vi "Example Two Stages.vi"() -> ()   [LabVIEW 2019]
uses:
  Class/Controller/Controller.lvclass
  <vilib>/Platform/TimedLoop/XDataNode/timing_clust.ctl
  <vilib>/Platform/TimedLoop/XDataNode/nitl_modes.ctl
  <vilib>/Platform/TimedLoop/XDataNode/wakeup.ctl
  <vilib>/platform/TimedLoop/XDataNode/XDataNode.xnode
  <vilib>/Platform/TimedLoop/XDataNode/XDNodeRunTimeDep.lvlib
panel:
  in  "Tab Control 2":enum32{"Motion", "Settings"}(tab)
  in  "Zero Output 2":bool
  in  "Go to Home 2":bool
  in  "Scan Right 2":bool
  in  "Scan Left 2":bool
  in  "Continue 2":bool
  in  "Stop 2":bool
  in  "Make Step Right 2":bool
  in  "Step Size \n[selected units] 2":dbl=1.0 format="%#.2f"
  in  "Make Step Left 2":bool
  in  "Desired Speed \n[1µm/s or 0,01deg /s] 2":dbl=10000.0 format="%#.2f"
  in  "Desired Position \n[selected units] 2":dbl format="%#.2f"
  in  "Find Index 2":bool
  in  "Reset 2":bool
  out "Desired Position\n[selected units] 2":dbl
  out "Encoder position \n[selected units] 2":dbl
  out "Waveform Chart 2":dbl(graph)=-0.078
  out "Status Info 2":T1
  out "StatusBits 2":T2
  out "Desired Position\n[selected units]":dbl
  out "Encoder position \n[selected units]":dbl
  in  "Tab Control":enum32{"Motion", "Settings"}(tab)
  in  "Zero Output":bool
  in  "Go to Home":bool
  in  "Scan Right":bool
  in  "Scan Left":bool
  in  "Continue":bool
  in  "Stop":bool
  in  "Make Step Right":bool
  in  "Step Size \n[selected units]":dbl=1.0 format="%#.2f"
  in  "Make Step Left":bool
  in  "Desired Speed \n[1µm/s or 0,01deg /s]":dbl=10000.0 format="%#.2f"
  in  "Desired Position \n[selected units]":dbl format="%#.2f"
  in  "Find Index":bool
  in  "Reset":bool
  out "error out":errorcluster
  in  "Working Units 2":string(combo)="1000000"
  in  "Working Units":string(combo)="1000000"
  out "StatusBits":T2
  out "Status Info":T1
  in  "Axis Resolution 2":string(combo)="312,5"
  in  "Axis Letter 2":string="Y"
  in  "Axis Resolution":string(combo)="312,5"
  in  "Axis Letter":string="X"
  in  "Baudrate":dbl=9600.0
  in  "COM Port":refnum<visa-resource-name>
  in  "Controller.lvclass":refnum<class "Controller.lvclass">
  out "Waveform Chart":dbl(graph)=-0.078
  in  "STOP PROGRAM":bool
  # "Visualization"
  # "Extra information"
  # "READ ME FIRST"
  # "Configuration"
  # "Stage 1"
  # "Driver 1"
  # "Stage 1"
  # "How to run:"
  # "BEFORE RUNNING:"
  # "1, Select COM Port"
  # "2. Select baudrate"
  # "3. For each axis:"
  # "3.1 Specify correct axis name (1 letter)"
  # "3.2 Specify correct resolution"
  # "4. Run VI"
  # "WHEN RUNNING, YOU HAVE TO FIRST PUSH \"FIND INDEX\" FOR EACH STAGE.\nThe stages will start moving and find its position. After that you can control the stages"
  # "Stage 2"
  # "NOTES: Do this only the first time"
  # "1. Replace the settings_default.txt file with\nthe file we provided on a USB stick."
  # "2.    Make sure there are no comments in the\nsettings_default.txt file. ONLY lines like: \"X:DPOS=100\" so NO \"%\" in front or at the end of the line."
  # "Position Information"
  # "STOP BUTTON"
  # "3.  In your settings_default.txt file:\nEvery line that contains SSPD or MSPD: multiply that value with:\n - 1000 for a lineair stage \n - 100 for a rotating stage"
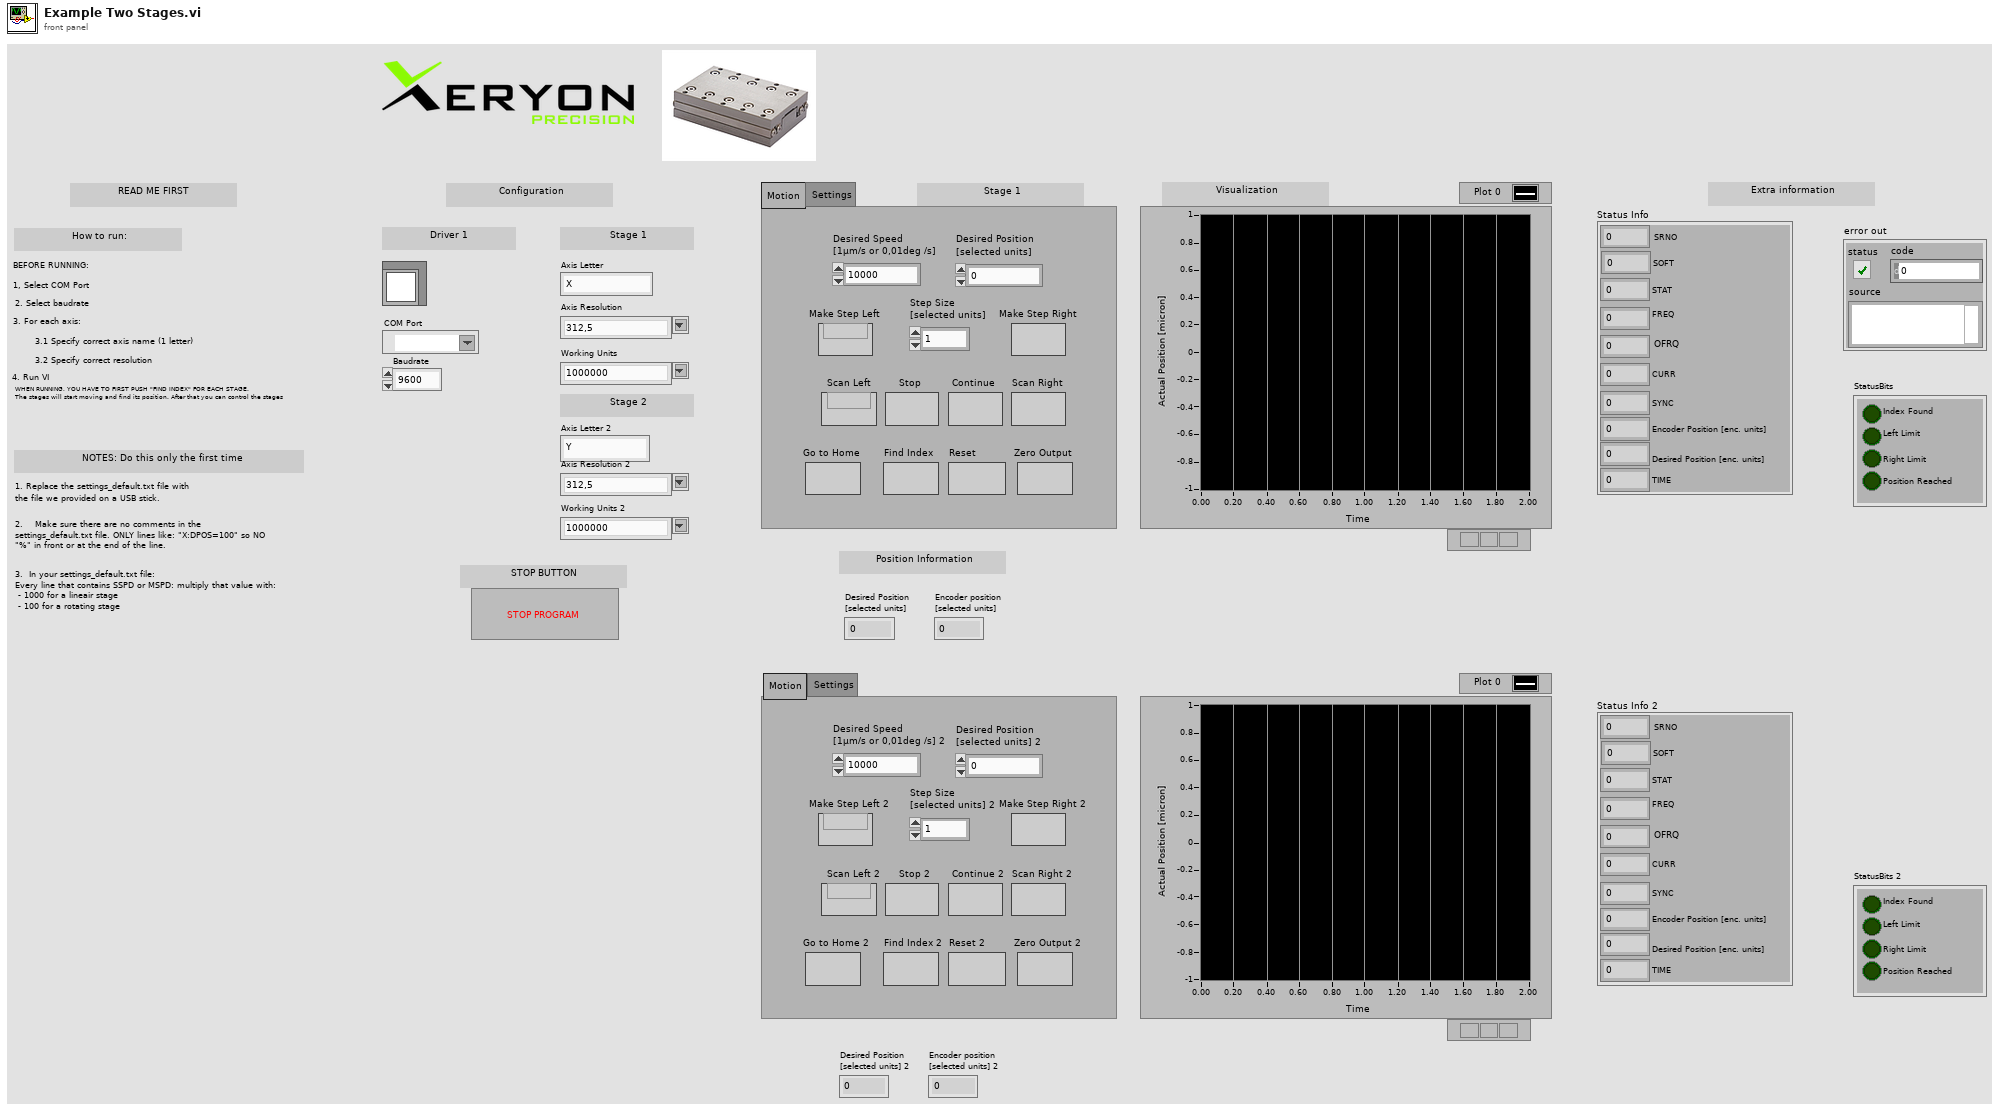
[diagram p1: front panel]
types:
  T1 = cluster{"SRNO":dbl, "SOFT":dbl, "STAT":dbl, "FREQ":dbl, "OFRQ":dbl, "CURR":dbl, "SYNC":dbl, "Encoder Position [enc. units]":dbl, "Desired Position [enc. units]":dbl, "TIME":dbl}
  T2 = cluster{"Index Found":bool, "Left Limit":bool, "Right Limit":bool, "Position Reached":bool}
  T3 = typedef "XDNodeRunTimeDep.lvlib/timing_clust.ctl" = cluster{"Expected End [f-1]":u64, "Actual End [f-1]":u64, "Finished Late? [f-1]":bool, "Expected End [i-1]":u64, "Actual End [i-1]":u64, "Finished Late? [i-1]":bool, "Expected Start [i]":u64, "Actual Start [i]":u64, "Expected Start [f]":u64, "Actual Start [f]":u64, "Source Name":string, "Structure Name":string, "Period":i64, "Deadline":i64, "Offset":i64, "Start":i64, "Priority":i32, "Timeout":i32, "Mode":T4, "Wakeup Reason":T5, "Error":errorcluster, "Source Type":string, "Secondary Source Type":string, "Global End Time":u64, "Global Start Time":u64, "Frame Duration":u64, "Iteration Duration":u64, "Assigned CPU":i32, "I/O Scan Engine Mode":u32}
  T4 = typedef "XDNodeRunTimeDep.lvlib/nitl_modes.ctl" = enum32{"No Change", "Process missed periods, maintain original phase", "Discard missed periods, maintain original phase", "Process missed periods, ignore original phase", "Discard missed periods, ignore original phase"}
  T5 = typedef "XDNodeRunTimeDep.lvlib/wakeup.ctl" = enum32{"Normal", "Aborted", "Asynchronous wakeup", "Timing source error", "Timed loop error", "Timeout"}
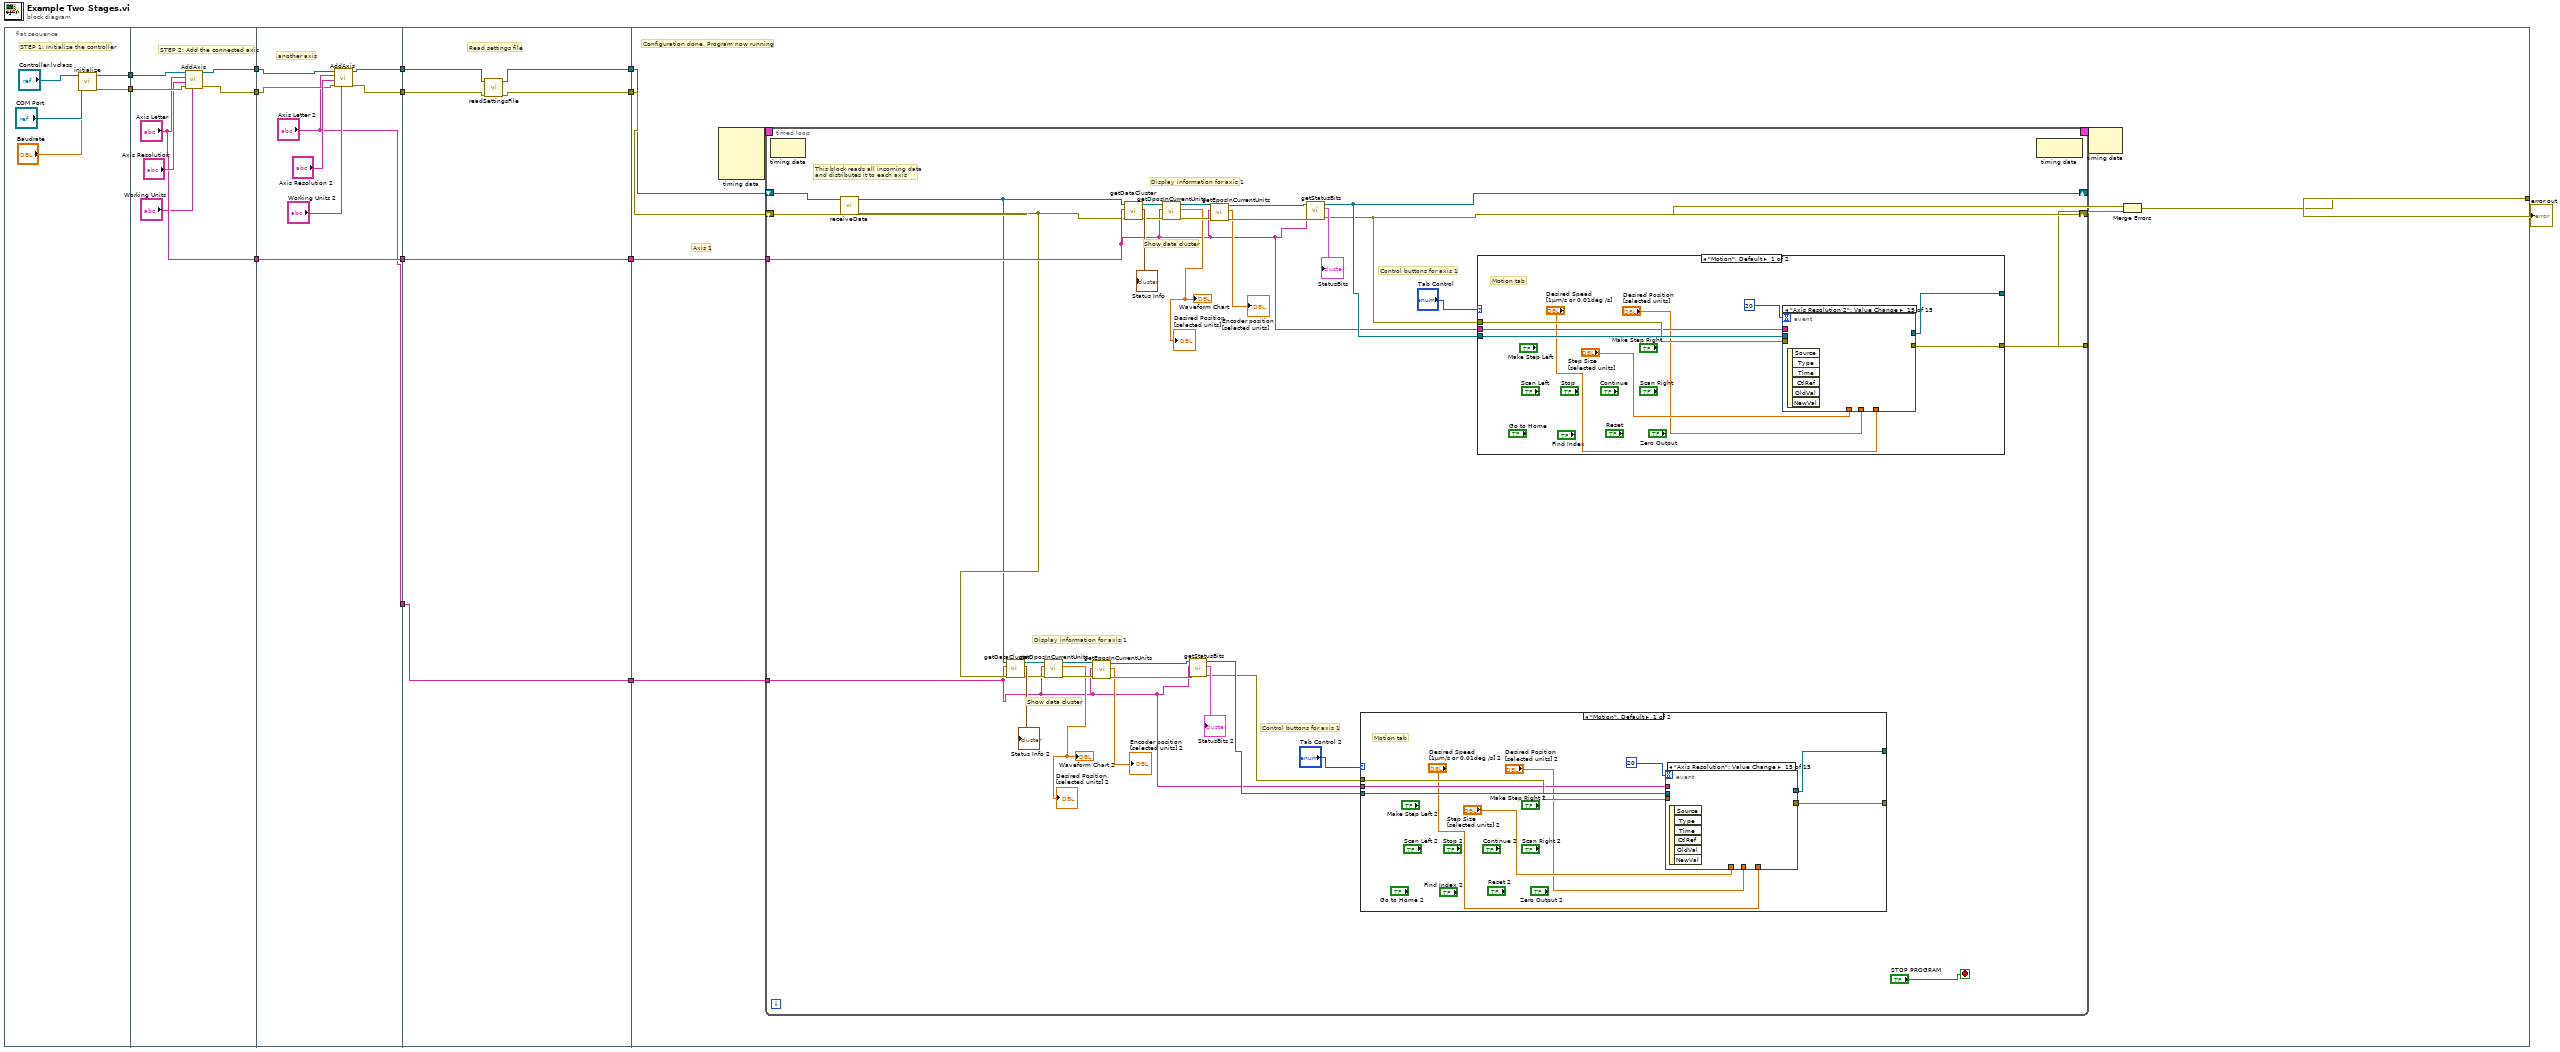
[diagram p0: block diagram]
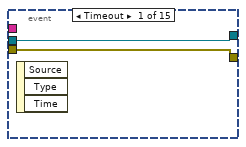
[diagram p2: hidden frame]
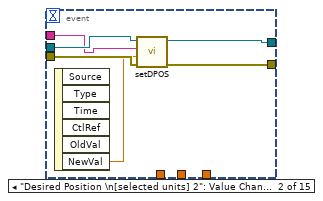
[diagram p3: hidden frame]
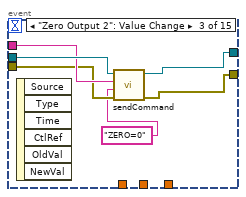
[diagram p4: hidden frame]
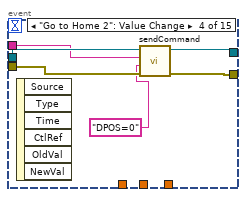
[diagram p5: hidden frame]
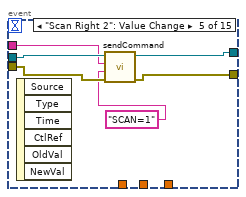
[diagram p6: hidden frame]
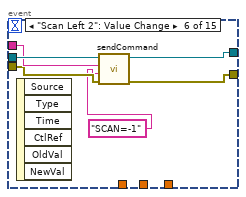
[diagram p7: hidden frame]
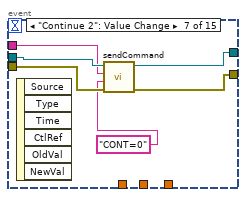
[diagram p8: hidden frame]
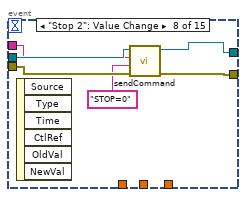
[diagram p9: hidden frame]
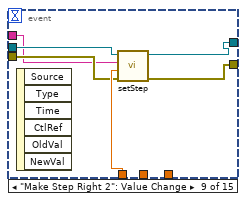
[diagram p10: hidden frame]
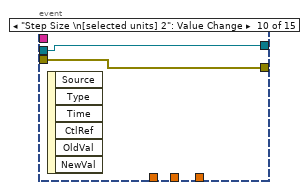
[diagram p11: hidden frame]
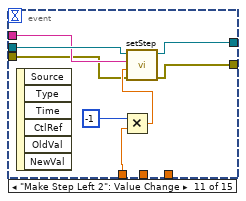
[diagram p12: hidden frame]
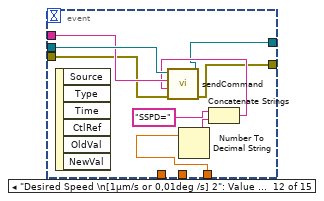
[diagram p13: hidden frame]
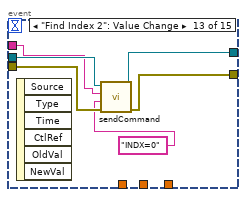
[diagram p14: hidden frame]
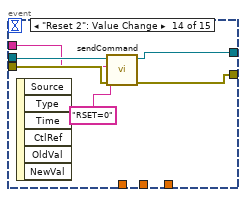
[diagram p15: hidden frame]
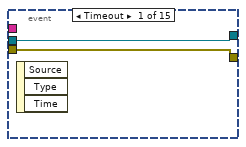
[diagram p17: hidden frame]
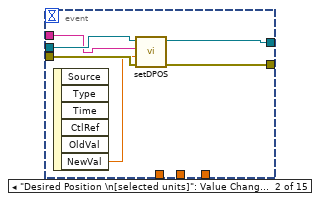
[diagram p18: hidden frame]
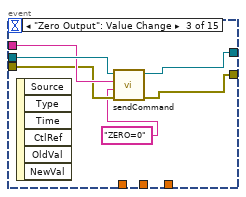
[diagram p19: hidden frame]
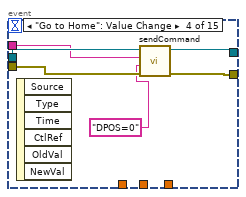
[diagram p20: hidden frame]
diagram:
  n1 = flat-sequence {
    tunnel: [w16] -> w14
    tunnel: [w15] -> w13
    tunnel: w14 -> [w26]
    tunnel: w13 -> [w25]
    tunnel: [w23] -> w12
    tunnel: [w22] -> w11
    tunnel: ["Axis Letter"] -> w10
    tunnel: w12 -> [w32]
    tunnel: w11 -> [w30]
    tunnel: [w34] -> w8
    tunnel: w10 -> [w34]
    tunnel: [w31] -> w6
    tunnel: [w29] -> w4
    tunnel: ["Axis Letter 2"] -> w2
    tunnel: w8 -> [w40]
    tunnel: [w40] -> w7
    tunnel: w6 -> [w39]
    tunnel: [w37] -> w5
    tunnel: w4 -> [w38]
    tunnel: [w36] -> w3
    tunnel: w2 -> [w35]
    tunnel: [w35] -> w1
    tunnel: w7 -> [w42]
    tunnel: w5 -> [w48]
    tunnel: w3 -> [w49]
    tunnel: [w44] -> w9
    tunnel: w1 -> [w41]
    frame #0 {
      # "STEP 1: Initialize the controller"
      n2 = call-dynamic "initialize.vi"("Baudrate"="Baudrate", "COM Port"="COM Port", "Controller in"="Controller.lvclass") -> ("error out"=w15:errorcluster, "Controller out"=w16:refnum<class "Controller.lvclass">)  [unwired: 7 in]
    }
    frame #1 {
      # "STEP 2: Add the connected axis"
      n3 = call-dynamic "AddAxis.vi"("Units"="Working Units", "error in (no error)"=w25, "Encoder Resolution"="Axis Resolution", "Axis Letter"="Axis Letter", "Controller in"=w26) -> ("error out"=w22:errorcluster, "Controller out"=w23:refnum<class "Controller.lvclass">)  [unwired: 5 in]
    }
    frame #2 {
      # "another axis"
      n4 = call-dynamic "AddAxis.vi"("Units"="Working Units 2", "error in (no error)"=w30, "Encoder Resolution"="Axis Resolution 2", "Axis Letter"="Axis Letter 2", "Controller in"=w32) -> ("error out"=w29:errorcluster, "Controller out"=w31:refnum<class "Controller.lvclass">)  [unwired: 5 in]
    }
    frame #3 {
      # "Read settings file"
      n5 = call-dynamic "readSettingsFile.vi"("error in (no error)"=w38, "Controller in"=w39) -> ("error out"=w36:errorcluster, "Controller out"=w37:refnum<class "Controller.lvclass">)  [unwired: 8 in]
    }
    frame #4 {
      # "Axis 1"
      # "Configuration done. Program now running"
      n6 = node-c288() -> (w47:T3)  [unwired: 4 in]
      n7 = timed-loop {
        shift-right: [w69] -> _
        shift-left: w48 -> [w83]
        tunnel: w42 -> [w67]
        shift-right: [w68] -> w45
        shift-left: w49 -> [w72]
        timing: w47 -> [_]
        timing-out: [_] -> w46
        tunnel: [w66] -> w43
        tunnel: w41 -> [w50]
        stop <- "STOP PROGRAM" stop-if-true
        # "Control buttons for axis 1"
        # "Display information for axis 1"
        # "Show data cluster"
        # "Control buttons for axis 1"
        # "Display information for axis 1"
        # "Show data cluster"
        # "This block reads all incoming data\nand distributes it to each axis"
        n8 = node-c288() -> ()  [unwired: 1 in, 1 out]
        n9 = call-dynamic "receiveData.vi"("error in (no error)"=w72, "Controller in"=w83) -> ("error out"=w52:errorcluster, "Controller out"=w51:refnum<class "Controller.lvclass">)  [unwired: 8 in]
        n10 = call-dynamic "getDataCluster.vi"("error in (no error)"=w52, "Axis Letter"=w50, "Controller in"=w51) -> ("error out"=w60:errorcluster, "Information"=→"Status Info 2":T1, "Controller out"=w63:refnum<class "Controller.lvclass">)  [unwired: 6 in]
        n11 = call-dynamic "getDposInCurrentUnits.vi"("error in (no error)"=w60, "Axis Letter"=w50, "Controller in"=w63) -> ("error out"=w59:errorcluster, "DPOS In Current Units"=→"Waveform Chart 2" →"Desired Position\n[selected units] 2":dbl, "Controller out"=w62:refnum<class "Controller.lvclass">)  [unwired: 6 in]
        n12 = call-dynamic "getEposInCurrentUnits.vi"("error in (no error)"=w59, "Axis Letter"=w50, "Controller in"=w62) -> ("error out"=w58:errorcluster, "EPOS In Current Units"=→"Encoder position \n[selected units] 2":dbl, "Controller out"=w61:refnum<class "Controller.lvclass">)  [unwired: 6 in]
        n13 = call-dynamic "getDataCluster.vi"("error in (no error)"=w52, "Axis Letter"=w67, "Controller in"=w51) -> ("error out"=w77:errorcluster, "Information"=→"Status Info":T1, "Controller out"=w80:refnum<class "Controller.lvclass">)  [unwired: 6 in]
        n14 = call-dynamic "getDposInCurrentUnits.vi"("error in (no error)"=w77, "Axis Letter"=w67, "Controller in"=w80) -> ("error out"=w76:errorcluster, "DPOS In Current Units"=→"Waveform Chart" →"Desired Position\n[selected units]":dbl, "Controller out"=w79:refnum<class "Controller.lvclass">)  [unwired: 6 in]
        n15 = call-dynamic "getStatusBits.vi"("error in (no error)"=w58, "Axis Letter"=w50, "Controller in"=w61) -> ("error out"=w53:errorcluster, "StatusBits"=→"StatusBits 2":T2, "Controller out"=w54:refnum<class "Controller.lvclass">)  [unwired: 6 in]
        n16 = call-dynamic "getEposInCurrentUnits.vi"("error in (no error)"=w76, "Axis Letter"=w67, "Controller in"=w79) -> ("error out"=w75:errorcluster, "EPOS In Current Units"=→"Encoder position \n[selected units]":dbl, "Controller out"=w78:refnum<class "Controller.lvclass">)  [unwired: 6 in]
        n17 = call-dynamic "getStatusBits.vi"("error in (no error)"=w75, "Axis Letter"=w67, "Controller in"=w78) -> ("error out"=w68:errorcluster, "StatusBits"=→"StatusBits":T2, "Controller out"=w69:refnum<class "Controller.lvclass">)  [unwired: 6 in]
        n18 = case shown="\"Motion\", Default" "Tab Control 2" {
          tunnel: w54 -> [w92 w174]
          tunnel: w53 -> [w91 w175]
          tunnel: [w90 w174] -> _
          tunnel: [w89 w175] -> _
          tunnel: w50 -> [w87 _]
          frame "Motion", Default {
            # "Motion tab"
            n19 = event shown="[14] \"Axis Resolution\": Value Change" {
              selector: _ -> [_ _ _ _ _ _ _ _ _ _ _ _ _ _ _]
              dyn-events: _ -> [_ _ _ _ _ _ _ _ _ _ _ _ _ _ _]
              timeout: 20 -> [_ _ _ _ _ _ _ _ _ _ _ _ _ _ _]
              tunnel: w92 -> [w94 w100 w106 w112 w118 w124 w130 w136 w140 w144 w150 w161 w167 w173 _]
              tunnel: w91 -> [w93 w99 w104 w110 w116 w122 w128 w134 w141 w143 w147 w159 w165 w172 _]
              tunnel: [w94 w97 w102 w107 w114 w120 w126 w132 w138 w144 w145 w153 w163 w169 _] -> w90
              tunnel: [w93 w98 w103 w109 w115 w121 w127 w133 w137 w143 w146 w154 w164 w168 _] -> w89
              tunnel: w87 -> [_ w95 w105 w111 w117 w123 w129 w135 w139 _ w149 w160 w166 w171 _]
              tunnel: "Step Size \n[selected units] 2" -> [_ _ _ _ _ _ _ _ w142 _ w151 _ _ _ _]
              tunnel: "Desired Position \n[selected units] 2" -> [_ _ _ _ _ _ _ _ _ _ _ _ _ _ _]
              tunnel: "Desired Speed \n[1µm/s or 0,01deg /s] 2" -> [_ _ _ _ _ _ _ _ _ _ _ w158 _ _ _]
              event Timeout {
                n20 = event-data() -> ()  [unwired: 1 in, 3 out]
              }
              event "Desired Position \n[selected units] 2": Value Change {
                n21 = event-data() -> ("NewVal"=w96:dbl)  [unwired: 1 in, 5 out]
                n22 = call-dynamic "setDPOS.vi"("error in (no error)"=w99, "DPOS In Current Units"=w96, "Axis Letter"=w95, "Controller in"=w100) -> ("error out"=w98:errorcluster, "Controller out"=w97:refnum<class "Controller.lvclass">)  [unwired: 6 in]
              }
              event "Zero Output 2": Value Change {
                n23 = event-data() -> ()  [unwired: 1 in, 6 out]
                n24 = call-dynamic "sendCommand.vi"("error in (no error)"=w104, "Command"="ZERO=0", "Axis Letter"=w105, "Controller in"=w106) -> ("error out"=w103:errorcluster, "Controller out"=w102:refnum<class "Controller.lvclass">)  [unwired: 6 in]
              }
              event "Go to Home 2": Value Change {
                n25 = event-data() -> ()  [unwired: 1 in, 6 out]
                n26 = call-dynamic "sendCommand.vi"("error in (no error)"=w110, "Command"="DPOS=0", "Axis Letter"=w111, "Controller in"=w112) -> ("error out"=w109:errorcluster, "Controller out"=w107:refnum<class "Controller.lvclass">)  [unwired: 6 in]
              }
              event "Scan Right 2": Value Change {
                n27 = event-data() -> ()  [unwired: 1 in, 6 out]
                n28 = call-dynamic "sendCommand.vi"("error in (no error)"=w116, "Command"="SCAN=1", "Axis Letter"=w117, "Controller in"=w118) -> ("error out"=w115:errorcluster, "Controller out"=w114:refnum<class "Controller.lvclass">)  [unwired: 6 in]
              }
              event "Scan Left 2": Value Change {
                n29 = event-data() -> ()  [unwired: 1 in, 6 out]
                n30 = call-dynamic "sendCommand.vi"("error in (no error)"=w122, "Command"="SCAN=-1", "Axis Letter"=w123, "Controller in"=w124) -> ("error out"=w121:errorcluster, "Controller out"=w120:refnum<class "Controller.lvclass">)  [unwired: 6 in]
              }
              event "Continue 2": Value Change {
                n31 = event-data() -> ()  [unwired: 1 in, 6 out]
                n32 = call-dynamic "sendCommand.vi"("error in (no error)"=w128, "Command"="CONT=0", "Axis Letter"=w129, "Controller in"=w130) -> ("error out"=w127:errorcluster, "Controller out"=w126:refnum<class "Controller.lvclass">)  [unwired: 6 in]
              }
              event "Stop 2": Value Change {
                n33 = event-data() -> ()  [unwired: 1 in, 6 out]
                n34 = call-dynamic "sendCommand.vi"("error in (no error)"=w134, "Command"="STOP=0", "Axis Letter"=w135, "Controller in"=w136) -> ("error out"=w133:errorcluster, "Controller out"=w132:refnum<class "Controller.lvclass">)  [unwired: 6 in]
              }
              event "Make Step Right 2": Value Change {
                n35 = event-data() -> ()  [unwired: 1 in, 6 out]
                n36 = call-dynamic "setStep.vi"("error in (no error)"=w141, "Step Value"=w142, "Axis Letter"=w139, "Controller in"=w140) -> ("error out"=w137:errorcluster, "Controller out"=w138:refnum<class "Controller.lvclass">)  [unwired: 6 in]
              }
              event "Step Size \n[selected units] 2": Value Change {
                n37 = event-data() -> ()  [unwired: 1 in, 6 out]
              }
              event "Make Step Left 2": Value Change {
                n38 = event-data() -> ()  [unwired: 1 in, 6 out]
                n39 = Multiply(x=-1, y=w151) -> (x*y=w148:dbl)
                n40 = call-dynamic "setStep.vi"("error in (no error)"=w147, "Step Value"=w148, "Axis Letter"=w149, "Controller in"=w150) -> ("error out"=w146:errorcluster, "Controller out"=w145:refnum<class "Controller.lvclass">)  [unwired: 6 in]
              }
              event "Desired Speed \n[1µm/s or 0,01deg /s] 2": Value Change {
                n41 = event-data() -> ()  [unwired: 1 in, 6 out]
                n42 = Number To Decimal String(number=w158) -> (decimal integer string=w156:string)  [unwired: 1 in]
                n43 = Concatenate Strings("SSPD=", w156) -> (w155:string)
                n44 = call-dynamic "sendCommand.vi"("error in (no error)"=w159, "Command"=w155, "Axis Letter"=w160, "Controller in"=w161) -> ("error out"=w154:errorcluster, "Controller out"=w153:refnum<class "Controller.lvclass">)  [unwired: 6 in]
              }
              event "Find Index 2": Value Change {
                n45 = event-data() -> ()  [unwired: 1 in, 6 out]
                n46 = call-dynamic "sendCommand.vi"("error in (no error)"=w165, "Command"="INDX=0", "Axis Letter"=w166, "Controller in"=w167) -> ("error out"=w164:errorcluster, "Controller out"=w163:refnum<class "Controller.lvclass">)  [unwired: 6 in]
              }
              event "Reset 2": Value Change {
                n47 = event-data() -> ()  [unwired: 1 in, 6 out]
                n48 = call-dynamic "sendCommand.vi"("error in (no error)"=w172, "Command"="RSET=0", "Axis Letter"=w171, "Controller in"=w173) -> ("error out"=w168:errorcluster, "Controller out"=w169:refnum<class "Controller.lvclass">)  [unwired: 6 in]
              }
              event "Axis Resolution": Value Change {
                n49 = event-data() -> ()  [unwired: 1 in, 6 out]
              }
            }
          }
          frame "Settings" {
          }
        }
        n50 = case shown="\"Motion\", Default" "Tab Control" {
          tunnel: w69 -> [w184 w266]
          tunnel: w68 -> [w183 w267]
          tunnel: [w182 w266] -> _
          tunnel: [w181 w267] -> w66
          tunnel: w67 -> [w179 _]
          frame "Motion", Default {
            # "Motion tab"
            n51 = event shown="[14] \"Axis Resolution 2\": Value Change" {
              selector: _ -> [_ _ _ _ _ _ _ _ _ _ _ _ _ _ _]
              dyn-events: _ -> [_ _ _ _ _ _ _ _ _ _ _ _ _ _ _]
              timeout: 20 -> [_ _ _ _ _ _ _ _ _ _ _ _ _ _ _]
              tunnel: w184 -> [w186 w192 w198 w204 w210 w216 w222 w228 w232 w236 w242 w253 w259 w265 _]
              tunnel: w183 -> [w185 w191 w196 w202 w208 w214 w220 w226 w233 w235 w239 w251 w257 w264 _]
              tunnel: [w186 w189 w194 w199 w206 w212 w218 w224 w230 w236 w237 w245 w255 w261 _] -> w182
              tunnel: [w185 w190 w195 w201 w207 w213 w219 w225 w229 w235 w238 w246 w256 w260 _] -> w181
              tunnel: w179 -> [_ w187 w197 w203 w209 w215 w221 w227 w231 _ w241 w252 w258 w263 _]
              tunnel: "Step Size \n[selected units]" -> [_ _ _ _ _ _ _ _ w234 _ w243 _ _ _ _]
              tunnel: "Desired Position \n[selected units]" -> [_ _ _ _ _ _ _ _ _ _ _ _ _ _ _]
              tunnel: "Desired Speed \n[1µm/s or 0,01deg /s]" -> [_ _ _ _ _ _ _ _ _ _ _ w250 _ _ _]
              event Timeout {
                n52 = event-data() -> ()  [unwired: 1 in, 3 out]
              }
              event "Desired Position \n[selected units]": Value Change {
                n53 = event-data() -> ("NewVal"=w188:dbl)  [unwired: 1 in, 5 out]
                n54 = call-dynamic "setDPOS.vi"("error in (no error)"=w191, "DPOS In Current Units"=w188, "Axis Letter"=w187, "Controller in"=w192) -> ("error out"=w190:errorcluster, "Controller out"=w189:refnum<class "Controller.lvclass">)  [unwired: 6 in]
              }
              event "Zero Output": Value Change {
                n55 = event-data() -> ()  [unwired: 1 in, 6 out]
                n56 = call-dynamic "sendCommand.vi"("error in (no error)"=w196, "Command"="ZERO=0", "Axis Letter"=w197, "Controller in"=w198) -> ("error out"=w195:errorcluster, "Controller out"=w194:refnum<class "Controller.lvclass">)  [unwired: 6 in]
              }
              event "Go to Home": Value Change {
                n57 = event-data() -> ()  [unwired: 1 in, 6 out]
                n58 = call-dynamic "sendCommand.vi"("error in (no error)"=w202, "Command"="DPOS=0", "Axis Letter"=w203, "Controller in"=w204) -> ("error out"=w201:errorcluster, "Controller out"=w199:refnum<class "Controller.lvclass">)  [unwired: 6 in]
              }
              event "Scan Right": Value Change {
                n59 = event-data() -> ()  [unwired: 1 in, 6 out]
                n60 = call-dynamic "sendCommand.vi"("error in (no error)"=w208, "Command"="SCAN=1", "Axis Letter"=w209, "Controller in"=w210) -> ("error out"=w207:errorcluster, "Controller out"=w206:refnum<class "Controller.lvclass">)  [unwired: 6 in]
              }
              event "Scan Left": Value Change {
                n61 = event-data() -> ()  [unwired: 1 in, 6 out]
                n62 = call-dynamic "sendCommand.vi"("error in (no error)"=w214, "Command"="SCAN=-1", "Axis Letter"=w215, "Controller in"=w216) -> ("error out"=w213:errorcluster, "Controller out"=w212:refnum<class "Controller.lvclass">)  [unwired: 6 in]
              }
              event "Continue": Value Change {
                n63 = event-data() -> ()  [unwired: 1 in, 6 out]
                n64 = call-dynamic "sendCommand.vi"("error in (no error)"=w220, "Command"="CONT=0", "Axis Letter"=w221, "Controller in"=w222) -> ("error out"=w219:errorcluster, "Controller out"=w218:refnum<class "Controller.lvclass">)  [unwired: 6 in]
              }
              event "Stop": Value Change {
                n65 = event-data() -> ()  [unwired: 1 in, 6 out]
                n66 = call-dynamic "sendCommand.vi"("error in (no error)"=w226, "Command"="STOP=0", "Axis Letter"=w227, "Controller in"=w228) -> ("error out"=w225:errorcluster, "Controller out"=w224:refnum<class "Controller.lvclass">)  [unwired: 6 in]
              }
              event "Make Step Right": Value Change {
                n67 = event-data() -> ()  [unwired: 1 in, 6 out]
                n68 = call-dynamic "setStep.vi"("error in (no error)"=w233, "Step Value"=w234, "Axis Letter"=w231, "Controller in"=w232) -> ("error out"=w229:errorcluster, "Controller out"=w230:refnum<class "Controller.lvclass">)  [unwired: 6 in]
              }
              event "Step Size \n[selected units]": Value Change {
                n69 = event-data() -> ()  [unwired: 1 in, 6 out]
              }
              event "Make Step Left": Value Change {
                n70 = event-data() -> ()  [unwired: 1 in, 6 out]
                n71 = Multiply(x=-1, y=w243) -> (x*y=w240:dbl)
                n72 = call-dynamic "setStep.vi"("error in (no error)"=w239, "Step Value"=w240, "Axis Letter"=w241, "Controller in"=w242) -> ("error out"=w238:errorcluster, "Controller out"=w237:refnum<class "Controller.lvclass">)  [unwired: 6 in]
              }
              event "Desired Speed \n[1µm/s or 0,01deg /s]": Value Change {
                n73 = event-data() -> ()  [unwired: 1 in, 6 out]
                n74 = Number To Decimal String(number=w250) -> (decimal integer string=w248:string)  [unwired: 1 in]
                n75 = Concatenate Strings("SSPD=", w248) -> (w247:string)
                n76 = call-dynamic "sendCommand.vi"("error in (no error)"=w251, "Command"=w247, "Axis Letter"=w252, "Controller in"=w253) -> ("error out"=w246:errorcluster, "Controller out"=w245:refnum<class "Controller.lvclass">)  [unwired: 6 in]
              }
              event "Find Index": Value Change {
                n77 = event-data() -> ()  [unwired: 1 in, 6 out]
                n78 = call-dynamic "sendCommand.vi"("error in (no error)"=w257, "Command"="INDX=0", "Axis Letter"=w258, "Controller in"=w259) -> ("error out"=w256:errorcluster, "Controller out"=w255:refnum<class "Controller.lvclass">)  [unwired: 6 in]
              }
              event "Reset": Value Change {
                n79 = event-data() -> ()  [unwired: 1 in, 6 out]
                n80 = call-dynamic "sendCommand.vi"("error in (no error)"=w264, "Command"="RSET=0", "Axis Letter"=w263, "Controller in"=w265) -> ("error out"=w260:errorcluster, "Controller out"=w261:refnum<class "Controller.lvclass">)  [unwired: 6 in]
              }
              event "Axis Resolution 2": Value Change {
                n81 = event-data() -> ()  [unwired: 1 in, 6 out]
              }
            }
          }
          frame "Settings" {
          }
        }
        n82 = node-c288() -> ()  [unwired: 1 in, 1 out]
      }
      n83 = node-c288(w46) -> ()  [unwired: 1 out]
      n84 = Merge Errors(w45, w43) -> (w44:errorcluster)
    }
  }
  "error out" <- w9
